vi "CFWSMetClient.vi"() -> (0 "Time Of Value (s)":dbl format="%#.1f", 1 "error out":errorcluster, 2 "RawPressure/mBar":dbl)   [LabVIEW 2018]
uses:
  <vilib>/httpClient/LabVIEWHTTPClient.lvlib
panel:
  out "ComputerTime":timestamp
  out "MetTimeStamp":timestamp
  out "data out":string
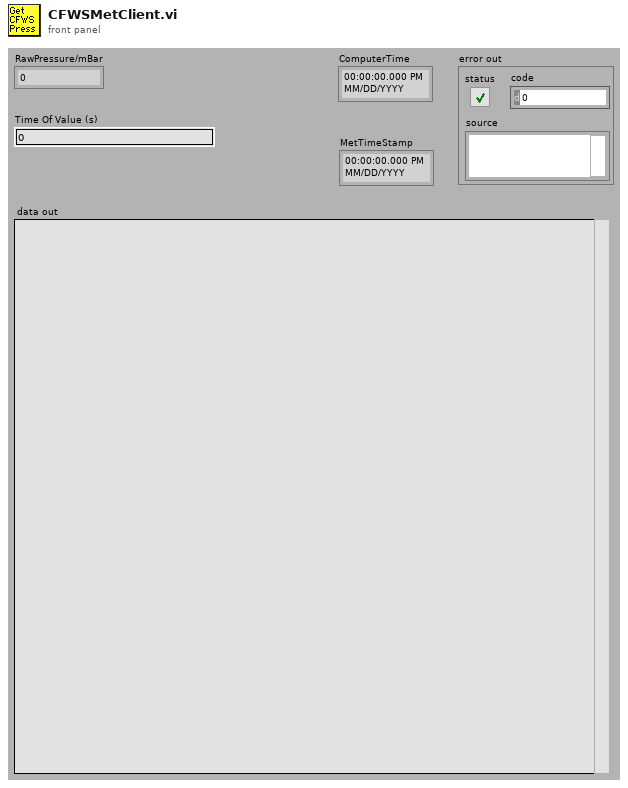
[diagram p1: front panel]
types:
  T1 = typedef "LabVIEWHTTPClient.lvlib/ClientHandle.ctl" = refnum<k1>
  T2 = cluster{"second":i32, "minute":i32, "hour":i32, "day of month":i32, "month":i32, "year":i32, "day of week":i32, "day of year":i32, "is DST":i32}
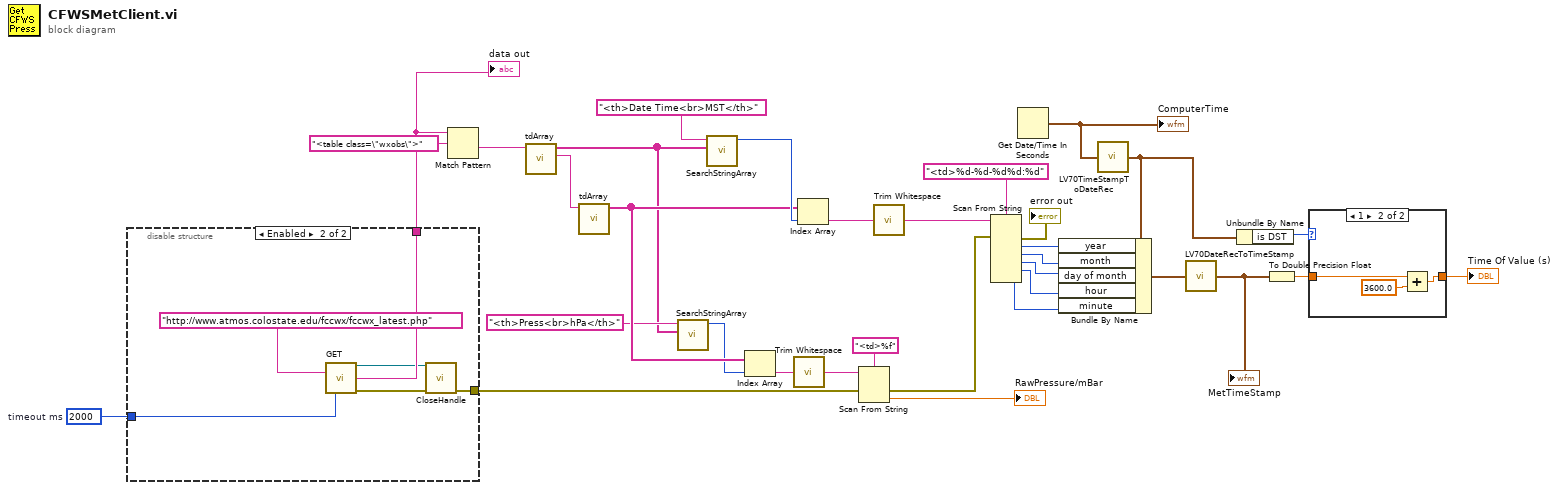
[diagram p0: block diagram]
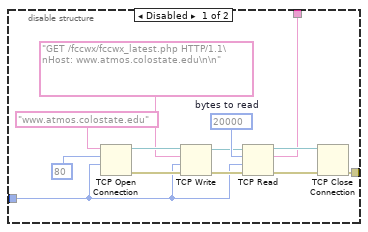
[diagram p2: hidden frame]
diagram:
  w1 = 2000  # timeout ms
  n1 = disable-structure shown="Enabled" {
    disable-tunnel: [w36 w50] -> w30
    disable-tunnel: [w35 w48] -> w2
    disable-tunnel: w1 -> [w34 w49]
    frame Disabled {
      w38 = 20000  # bytes to read
      n2 = TCP Open Connection(address="www.atmos.colostate.edu", remote port or service name=u16 80 ("remote port"), timeout ms (60000)=w34) -> (connection ID=w43:refnum<k5>, error out=w41:errorcluster)  [unwired: 1 in, 1 out]
      n3 = TCP Write(connection ID=w43, data in="GET /fccwx/fccwx_latest.php HTTP/1.1\nHost: www.atmos.colostate.edu\n\n", error in (no error)=w41, 9:w34) -> (connection ID out=w37:refnum<k5>, error out=w40:errorcluster)  [unwired: 1 out]
      n4 = TCP Read(connection ID=w37, bytes to read=w38, error in (no error)=w40, 9:w34) -> (connection ID out=w39:refnum<k5>, data out=w36:string, error out=w35:errorcluster)  [unwired: 1 out]
      n5 = TCP Close Connection(connection ID=w39) -> ()  [unwired: 1 in, 3 out]
    }
    frame Enabled {
      n6 = call <vilib>:"GET.vi"("url"="http://www.atmos.colostate.edu/fccwx/fccwx_latest.php", "timeout (10000)"=w49) -> ("client handle out"=w46:T1, "body"=w50:string, "error out"=w47:errorcluster)  [unwired: 10 in, 1 out]
      n7 = call <vilib>:"CloseHandle.vi"("client handle"=w46, "error in (no error)"=w47) -> ("error out"=w48:errorcluster)  [unwired: 13 in]
    }
  }
  "data out" <- w30
  n8 = Match Pattern(string=w30, regular expression="<table class=\"wxobs\">") -> (after substring=w28:string)  [unwired: 4 out]
  n9 = call "tdArray.vi"("tableIn"=w28) -> ("remainingTable"=w9:string, "firstRow"=w6:string[])  [unwired: 9 in]
  n10 = call "tdArray.vi"("tableIn"=w9) -> ("firstRow"=w8:string[])  [unwired: 9 in, 1 out]
  n11 = call "SearchStringArray.vi"("stringArray"=w6, "String"="<th>Press<br>hPa</th>") -> ("foundIndex"=w5:i32)  [unwired: 9 in]
  n12 = call "SearchStringArray.vi"("stringArray"=w6, "String"="<th>Date Time<br>MST</th>") -> ("foundIndex"=w27:i32)  [unwired: 9 in]
  n13 = Index Array(array=w8, index=w5) -> (element=w15:string)
  n14 = call <vilib>:"Trim Whitespace.vi"("string"=w15) -> ("trimmed string"=w16:string)  [unwired: 1 in]
  n15 = Index Array(array=w8, index=w27) -> (element=w24:string)
  n16 = Scan From String(format string="<td>%f", input string=w16, error in=w2) -> (error out=w4:errorcluster, output 1=→"RawPressure/mBar":dbl)  [unwired: 1 in, 3 out]
  n17 = call <vilib>:"Trim Whitespace.vi"("string"=w24) -> ("trimmed string"=w17:string)  [unwired: 1 in]
  n18 = Scan From String(format string="<td>%d-%d-%d%d:%d", input string=w17, error in=w4) -> (error out=→"error out":errorcluster, output 1=w23:i32, output 2=w22:i32, output 3=w21:i32, output 4=w20:i32, output 5=w19:i32)  [unwired: 1 in, 7 out]
  n19 = Get Date/Time In Seconds() -> (seconds since 1Jan1904=w10:timestamp)
  "ComputerTime" <- w10
  n20 = call <vilib>:"LV70TimeStampToDateRec.vi"("time stamp"=w10) -> ("date time rec"=w12:T2)
  n21 = Bundle By Name(cluster=w12, "year"=w23, "month"=w22, "day of month"=w21, "hour"=w20, "minute"=w19) -> (w18:T2)
  n22 = call <vilib>:"LV70DateRecToTimeStamp.vi"("date time rec"=w18) -> ("Time Stamp"=w11:timestamp)
  "MetTimeStamp" <- w11
  n23 = Unbundle By Name(w12) -> ("is DST"=w33:i32)
  n24 = To Double Precision Float(number=w11) -> (double precision float=w32:dbl)
  n25 = case shown="1" w33 {
    tunnel: w32 -> [w52 w55]
    tunnel: [w52 w53] -> w31
    frame 0, Default {
    }
    frame 1 {
      n26 = Add(x=w55, y=3600.0) -> (x+y=w53:dbl)
    }
  }
  "Time Of Value (s)" <- w31
